vi "EdgeDetection.vi"() -> ()   [LabVIEW 2017]
uses:
  <vilib>/vision/NI_Vision_Development_Module.lvlib
panel:
  in  "Method":T1(ring)=enum."Sobel"
  in  "Threshold Value":sgl=90.0
  out "Image":T2(plugin-control)
  out "error out":errorcluster
  in  "error in (no error)":errorcluster
  in  "File Path":path
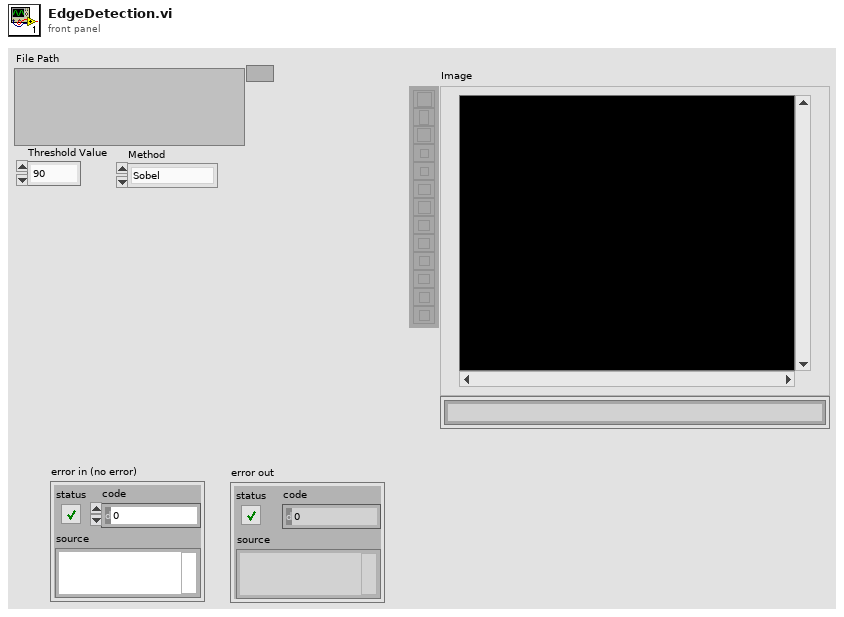
[diagram p1: front panel]
types:
  T1 = enum32{"Differentiation", "Gradient", "Prewitt", "Roberts", "Sigma", "Sobel"}
  T2 = typedef "IMAQ Image.ctl" = refnum<image>
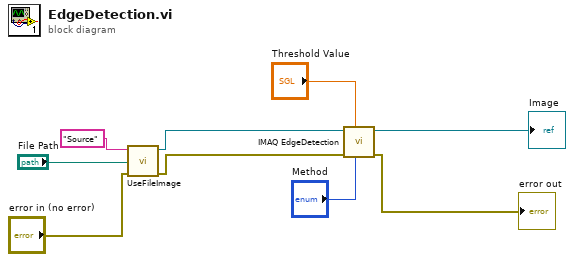
[diagram p0: block diagram]
diagram:
  n1 = call "UseFileImage.vi"("error in (no error)"="error in (no error)", "File Path"="File Path", "Image Name"="Source") -> ("error out"=w5:errorcluster, "Original Image"=w6:T2)  [unwired: 7 in]
  n2 = call "IMAQ EdgeDetection"("Method"="Method", "Threshold Value"="Threshold Value", "error in (no error)"=w5, "Image Src"=w6) -> ("error out"=→"error out":errorcluster, "Image Dst Out"=→"Image":T2)  [unwired: 6 in]
